vi "_시리얼 데이타 수신.vi"(3 "전송 문자열":string="*IDN?", 4 "ErrIn":bool=TRUE, 5 "시리얼 포트":refnum<visa-resource-name>="COM3") -> (0 "수신 문자열":string, 1 "Processing TIme(ms)":u32=12, 2 "수신 실패(T)":bool)   [LabVIEW 2015]
panel:
  out "Error":string="*IDN?"
  out "웨이브폼 차트":u32(graph)
  out "에러 출력":errorcluster={"status"=FALSE, "code"=1073676294, "source"="_시리얼 데이타 수신.vi 안에 VISA 읽기"}
  out "수신 문자열 버퍼":string
  out "최종 수신 문자열":string
  out "수신 타이머 값":u32=2566765
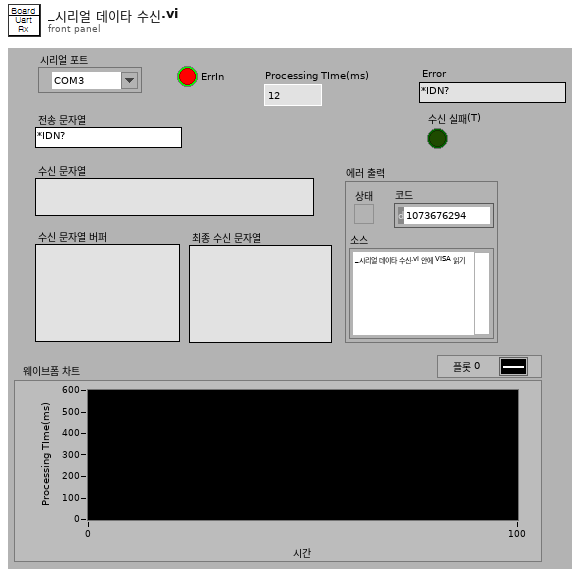
[diagram p1: front panel]
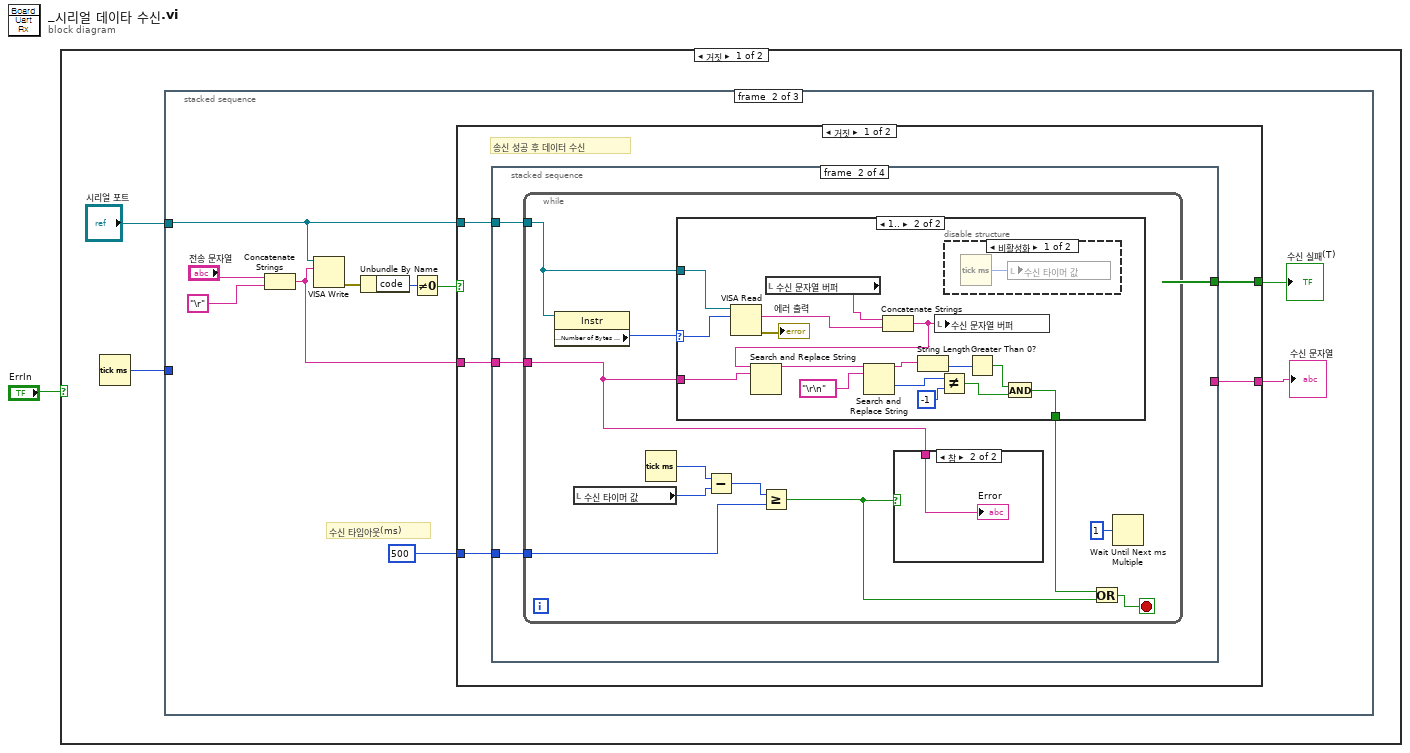
[diagram p0: block diagram]
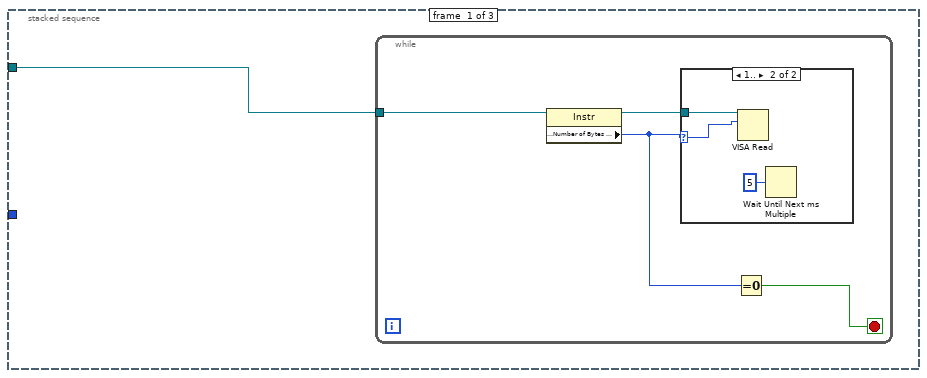
[diagram p2: hidden frame]
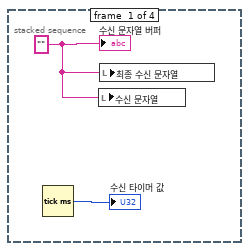
[diagram p4: hidden frame]
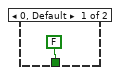
[diagram p6: hidden frame]
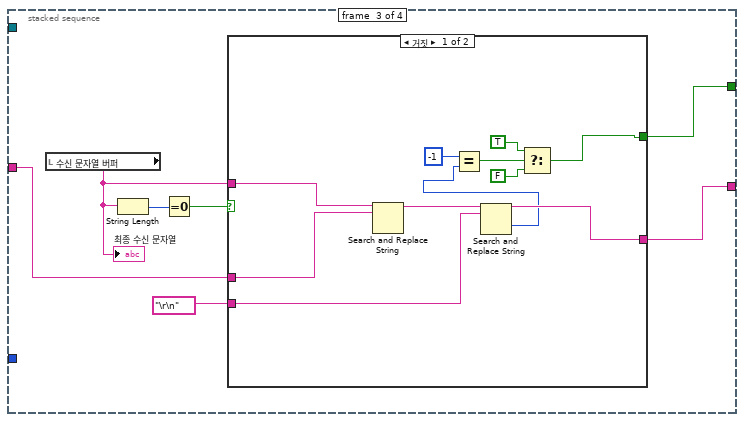
[diagram p8: hidden frame]
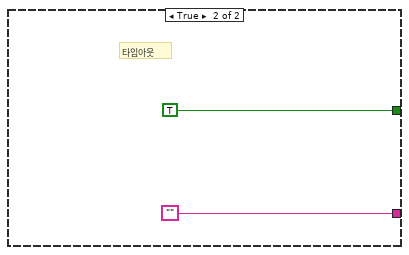
[diagram p9: hidden frame]
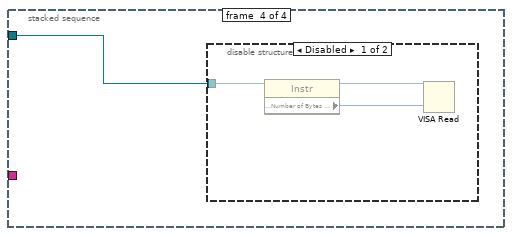
[diagram p10: hidden frame]
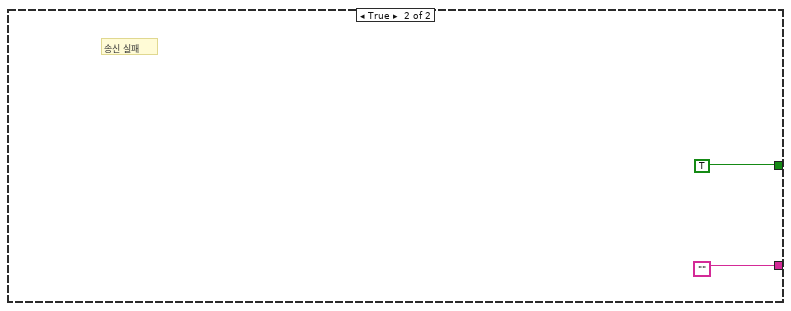
[diagram p12: hidden frame]
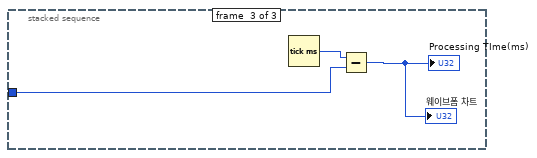
[diagram p13: hidden frame]
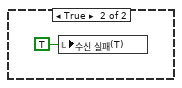
[diagram p14: hidden frame]
diagram:
  n1 = case shown="거짓" "ErrIn" {
    frame False {
      n2 = Tick Count (ms)() -> (millisecond timer value=w2:u32)
      n3 = stacked-sequence {
        tunnel: "시리얼 포트" -> [w4 w12 _]
        tunnel: w2 -> [_ _ w89]
        frame #0 {
          n4 = while {
            tunnel: w4 -> [w7]
            stop <- w6 stop-if-true
            n5 = property class="Instr"(reference=w7) -> (reference out=w8:refnum<visa-resource-name>, "Serial Settings:Number of Bytes at Serial Port"=w5:u32)  [unwired: 1 in, 1 out]
            n6 = case shown="1.." w5 {
              selector: w5 -> [_ w10]
              tunnel: w8 -> [_ w11]
              frame 0, Default {
              }
              frame 1.. {
                n7 = VISA Read(VISA resource name=w11, byte count=w10) -> ()  [unwired: 1 in, 4 out]
                n8 = Wait Until Next ms Multiple(millisecond multiple=u32 5 ("ms 배수")) -> ()  [unwired: 1 out]
              }
            }
            n9 = Equal To 0?(x=w5) -> (x = 0?=w6:bool)
          }
        }
        frame #1 {
          # "수신 타임아웃(ms)"
          n10 = Concatenate Strings("전송 문자열", "\r") -> (w13:string)
          n11 = VISA Write(VISA resource name=w12, write buffer=w13) -> (error out=w21:errorcluster)  [unwired: 1 in, 2 out]
          n12 = Unbundle By Name(w21) -> ("code"=w20:i32)
          n13 = Not Equal To 0?(x=w20) -> (x != 0?=w19:bool)
          n14 = case shown="거짓" w19 {
            tunnel: [w23 ""] -> w16
            tunnel: [w24 TRUE] -> w18
            tunnel: w12 -> [w26 _]
            tunnel: 500 -> [w25 _]
            tunnel: w13 -> [w22 _]
            frame False {
              # "송신 성공 후 데이터 수신"
              n15 = stacked-sequence {
                tunnel: w26 -> [_ w31 _ w82]
                tunnel: w25 -> [_ w30 _ _]
                tunnel: [_ _ w68 _] -> w24
                tunnel: [_ _ w67 _] -> w23
                tunnel: w22 -> [_ w29 w62 _]
                frame #0 {
                  w27 = "" ("수신 문자열")
                  n16 = Tick Count (ms)() -> (millisecond timer value=→"수신 타이머 값":u32)
                  n17 = local write "수신 문자열"(w27) -> ()
                  n18 = local write "최종 수신 문자열"(w27) -> ()
                  "수신 문자열 버퍼" <- w27
                }
                frame #1 {
                  n19 = while {
                    tunnel: w31 -> [w42]
                    tunnel: w30 -> [w38]
                    tunnel: w29 -> [w32]
                    stop <- w37 stop-if-true
                    n20 = property class="Instr"(reference=w42) -> ("Serial Settings:Number of Bytes at Serial Port"=w34:u32)  [unwired: 1 in, 2 out]
                    n21 = local read "수신 타이머 값"() -> (w40:u32)
                    n22 = Tick Count (ms)() -> (millisecond timer value=w41:u32)
                    n23 = case shown="1.." w34 {
                      selector: w34 -> [_ w46]
                      tunnel: w42 -> [_ w59]
                      tunnel: [FALSE w52] -> w36
                      tunnel: w32 -> [_ w50]
                      frame 0, Default {
                      }
                      frame 1.. {
                        n24 = VISA Read(VISA resource name=w59, byte count=w46) -> (read buffer=w58:string, error out=→"에러 출력":errorcluster)  [unwired: 1 in, 2 out]
                        n25 = local read "수신 문자열 버퍼"() -> (w60:string)
                        n26 = Concatenate Strings(w60, w58) -> (w51:string)
                        n27 = Search and Replace String(input string=w51, search string=w50) -> (result string=w48:string)  [unwired: 6 in, 3 out]
                        n28 = Search and Replace String(input string=w48, search string="\r\n") -> (result string=w56:string, offset past replacement=w47:i32)  [unwired: 6 in, 2 out]
                        n29 = String Length(string=w56) -> (length=w55:i32)
                        n30 = local write "수신 문자열 버퍼"(w51) -> ()
                        n31 = Not Equal?(x=w47, y=-1) -> (x != y?=w54:bool)
                        n32 = disable-structure shown="비활성화" {
                          frame Disabled {
                            n33 = Tick Count (ms)() -> (millisecond timer value=w61:u32)
                            n34 = local write "수신 타이머 값"(w61) -> ()
                          }
                          frame Enabled {
                          }
                        }
                        n35 = Greater Than 0?(x=w55) -> (x > 0?=w53:bool)
                        n36 = And(x=w53, y=w54) -> (x .and. y?=w52:bool)
                      }
                    }
                    n37 = Subtract(x=w41, y=w40) -> (x-y=w39:u32)
                    n38 = Greater Or Equal?(x=w39, y=w38) -> (x >= y?=w33:bool)
                    n39 = case shown="참" w33 {
                      tunnel: w32 -> [_ w43]
                      frame False {
                      }
                      frame True {
                        "Error" <- w43
                      }
                    }
                    n40 = Or(x=w36, y=w33) -> (x .or. y?=w37:bool)
                    n41 = Wait Until Next ms Multiple(millisecond multiple=u32 1 ("ms 배수")) -> ()  [unwired: 1 out]
                  }
                }
                frame #2 {
                  n42 = local read "수신 문자열 버퍼"() -> (w63:string)
                  "최종 수신 문자열" <- w63
                  n43 = String Length(string=w63) -> (length=w65:i32)
                  n44 = Equal To 0?(x=w65) -> (x = 0?=w66:bool)
                  n45 = case shown="거짓" w66 {
                    tunnel: [w76 TRUE] -> w68
                    tunnel: [w79 ""] -> w67
                    tunnel: "\r\n" -> [w70 _]
                    tunnel: w63 -> [w73 _]
                    tunnel: w62 -> [w72 _]
                    frame False {
                      n46 = Search and Replace String(input string=w73, search string=w72) -> (result string=w71:string)  [unwired: 6 in, 3 out]
                      n47 = Search and Replace String(input string=w71, search string=w70) -> (result string=w79:string, offset past replacement=w69:i32)  [unwired: 6 in, 2 out]
                      n48 = Equal?(x=-1, y=w69) -> (x = y?=w77:bool)
                      n49 = Select(t=TRUE, s=w77, f=FALSE) -> (s? t:f=w76:bool)
                    }
                    frame True {
                      # "타임아웃"
                    }
                  }
                }
                frame #3 {
                  n50 = disable-structure shown="Disabled" {
                    disable-tunnel: w82 -> [w83 _]
                    frame Disabled {
                      n51 = property class="Instr"(reference=w83) -> (reference out=w84:refnum<visa-resource-name>, "Serial Settings:Number of Bytes at Serial Port"=w85:u32)  [unwired: 1 in, 1 out]
                      n52 = VISA Read(VISA resource name=w84, byte count=w85) -> ()  [unwired: 1 in, 4 out]
                    }
                    frame Enabled {
                    }
                  }
                }
              }
            }
            frame True {
              # "송신 실패"
            }
          }
          "수신 문자열" <- w16
          "수신 실패(T)" <- w18
        }
        frame #2 {
          n53 = Tick Count (ms)() -> (millisecond timer value=w90:u32)
          n54 = Subtract(x=w90, y=w89) -> (x-y=→"Processing TIme(ms)" →"웨이브폼 차트":u32)
        }
      }
    }
    frame True {
      n55 = local write "수신 실패(T)"(TRUE ("수신 실패(T)")) -> ()
    }
  }
